vi "Show Series Launched Panel.vi"(8 "error in":errorcluster, 10 "Panel Ident":string, 11 "Study Actor in":refnum<class "Study Actor.lvclass">) -> (0 "error out":errorcluster, 3 "Study Actor out":refnum<class "Study Actor.lvclass">)   [LabVIEW 2024, in "Study Actor.lvlib" / "Study Actor.lvclass"]
uses:
  Study Actor.lvclass
  Study Actor.lvclass/Study Actor.ctl
  Series/ISeries Actor/ISeries Actor Messages/Show Nested Panel Msg/Show Nested Panel Msg.lvclass/Show Nested Panel Msg.ctl
  <vilib>/ActorFramework/Message Enqueuer/Message Enqueuer.lvclass/Message Enqueuer.ctl
  IStudy Actor Messages/Log Target Msg/Log Target Msg.lvclass/Log Target Msg.ctl
  <vilib>/ActorFramework/Message Enqueuer/Enqueue.vi
  Series/ISeries Actor/ISeries Actor Messages/Show Nested Panel Msg/Show Nested Panel Msg.lvclass
  C:/Program Files/National Instruments/LabVIEW 2024/vi.lib/ActorFramework/Message/Message.lvclass
  IStudy Actor Messages/Log Target Msg/Log Target Msg.lvclass
  <vilib>/Utility/LVClass/Get LV Class Name.vi
  <resource>/AFDebug/Generate Trace for Message.vi
  <vilib>/ActorFramework/Message Priority Queue/Priority Enqueue.vi
  <vilib>/ActorFramework/Actor/Actor.lvclass
  C:/Program Files/National Instruments/LabVIEW 2024/vi.lib/MGI/Panel Manager/Panel Actor/Panel Actor/Panel Actor.lvclass
  C:/Program Files/National Instruments/LabVIEW 2024/vi.lib/ActorFramework/Actor/Actor.lvclass
  D:/git/HAL/MAL/Study/Study Actor/Study Actor/Study Actor.lvclass
  D:/git/HAL/MAL/Study/Study Actor/IStudy Actor/IStudy Actor.lvclass
  C:/Program Files/National Instruments/LabVIEW 2024/vi.lib/ni/Actors/Network Endpoint Actors/Nested Endpoint Caller/Nested Endpoint Caller/Nested Endpoint Caller.lvclass
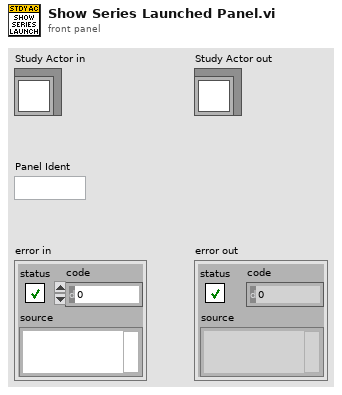
[diagram p1: front panel]
types:
  T1 = map{string, refnum<class "Message Enqueuer.lvclass">}
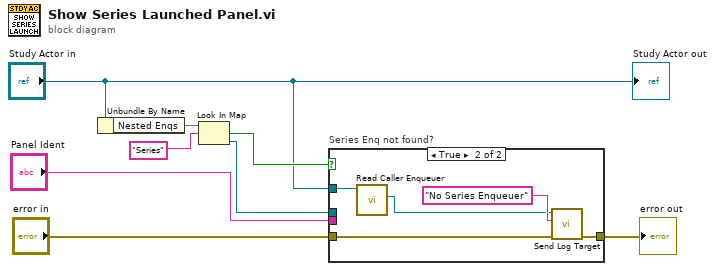
[diagram p0: block diagram]
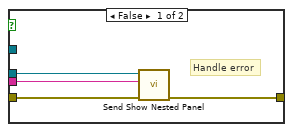
[diagram p2: hidden frame]
diagram:
  n1 = Unbundle By Name("Study Actor in") -> ("Nested Enqs"=w8:T1)
  n2 = Look In Map(map=w8, key="Series") -> (key not found?=w2:bool, value=w4:refnum<class "Message Enqueuer.lvclass">)  [unwired: 1 in]
  n3 = case "Series Enq not found?" shown="True" w2 {
    tunnel: "error in" -> [w12 w17]
    tunnel: [w11 w16] -> w5
    tunnel: w4 -> [w10 _]
    tunnel: "Panel Ident" -> [w9 _]
    tunnel: "Study Actor in" -> [_ w14]
    frame False {
      # "Handle error"
      n4 = call "Send Show Nested Panel.vi"("error in (no error)"=w12, "Panel Ident"=w9, "Message Enqueuer"=w10) -> ("error out"=w11:errorcluster)  [unwired: 7 in, 1 out]
    }
    frame True {
      n5 = call <vilib>:"Read Caller Enqueuer.vi"("Actor"=w14) -> ("Caller Enqueuer"=w13:refnum<class "Message Enqueuer.lvclass">)  [unwired: 10 in]
      n6 = call "Send Log Target.vi"("error in (no error)"=w17, "Entry"="No Series Enqueuer", "Message Enqueuer"=w13) -> ("error out"=w16:errorcluster)  [unwired: 7 in, 1 out]
    }
  }
  "error out" <- w5
  "Study Actor out" <- "Study Actor in"
